vi "Create.vi"(0 "Type":string, 5 "Event":string, 7 "Target":string) -> (4 "Termination":refnum<class "Termination.lvclass">)   [LabVIEW 2020, in "Termination.lvclass"]
uses:
  Termination.lvclass
  Typedefs/Tosca-Termination Condition Action.ctl
  Typedefs/Tosca-Event Type.ctl
  Termination.lvclass/Termination.ctl
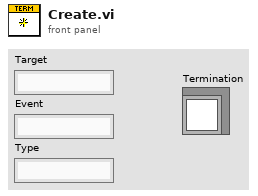
[diagram p1: front panel]
types:
  T1 = typedef "Tosca-Termination Condition Action.ctl" = enum16{"End state", "Complete state", "TTL only"}
  T2 = typedef "Tosca-Event Type.ctl" = enum16{"Normal", "CS+", "CS-"}
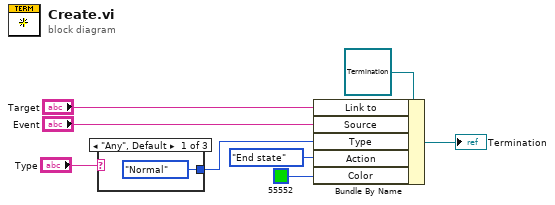
[diagram p0: block diagram]
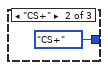
[diagram p2: hidden frame]
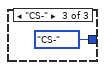
[diagram p3: hidden frame]
diagram:
  n1 = case shown="\"Any\", Default" "Type" {
    tunnel: [Tosca-Event_Type."Normal" ("Serialized.Type") Tosca-Event_Type."CS+" ("Serialized.Type") Tosca-Event_Type."CS-" ("Serialized.Type")] -> w4
    frame "Any", Default {
    }
    frame "CS+" {
    }
    frame "CS-" {
    }
  }
  n2 = Bundle By Name(cluster=refnum<class "Termination.lvclass"> refnum ("Termination"), "Link to"="Target", "Source"="Event", "Type"=w4, "Action"=Tosca-Termination_Condition_Action."End state" ("Serialized.Action"), "Color"=u32 55552) -> (→"Termination":refnum<class "Termination.lvclass">)
